vi "EdgeDetect.vi"   [LabVIEW 2019]
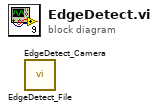
[diagram p0: block diagram]
diagram:
  n1 = call <userlib>:"EdgeDetect_File.vi"() -> ()  [unwired: 12 in, 4 out]
  n2 = call <userlib>:"EdgeDetect_Camera.vi"() -> ()  [unwired: 12 in, 4 out]
